vi "Not a Window Refnum.vi"() -> (0 "Not a Window Refnum":T1)   [LabVIEW 2020, in "Win Util New.lvlib"]
uses:
  Win Util New.lvlib
  Window Refnum.ctl
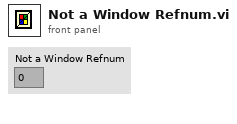
[diagram p1: front panel]
types:
  T1 = typedef "Win Util New.lvlib/Window Refnum.ctl" = u64
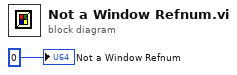
[diagram p0: block diagram]
diagram:
  "Not a Window Refnum" <- T1 0 ("Not a Window Refnum")
